vi "SpikeMIDI.vi"() -> ()   [LabVIEW 2022 SP3]
uses:
  _LVsubs/MakeYourOwn/Serial_Port.xctl
  _LVsubs/MakeYourOwn/Code.xctl
  _LVsubs/MakeYourOwn/File Tree.xctl
panel:
  in  "sensor 6":u16(ring)=1 items=["", "Touch Sensor", "Color Sensor", "Force and Distance", "Color and Distance", "Force and Motor", "Color and Motor"]
  in  "Port 7":string="A"
  in  "port 6":string="F"
  in  "six notes":bool
  in  "note (input a number) 6":string="70"
  in  "sensor 5":u16(ring)=1 items=["", "Touch Sensor", "Color Sensor", "Force and Distance", "Color and Distance", "Force and Motor", "Color and Motor"]
  in  "Port 6":string="B"
  in  "port 5":string="E"
  in  "five notes":bool
  in  "note (input a number) 5":string="70"
  in  "sensor 4":u16(ring)=1 items=["", "Touch Sensor", "Color Sensor", "Force and Distance", "Color and Distance", "Force and Motor", "Color and Motor"]
  in  "Port 5":string="C"
  in  "port 4":string="D"
  in  "four notes":bool
  in  "note (input a number) 4":string="70"
  in  "sensor 3":u16(ring)=1 items=["", "Touch Sensor", "Color Sensor", "Force and Distance", "Color and Distance", "Force and Motor", "Color and Motor"]
  in  "Port 4":string="D"
  in  "port 3":string="C"
  in  "three notes":bool
  in  "note (input a number) 3":string="70"
  in  "sensor 2":u16(ring)=1 items=["", "Touch Sensor", "Color Sensor", "Force and Distance", "Color and Distance", "Force and Motor", "Color and Motor"]
  in  "Port 3":string="E"
  in  "port 2":string="B"
  in  "two notes":bool
  in  "note (input a number) 2":string="70"
  in  "Port 2":string="F"
  in  "Port":string="A"
  in  "note (input a number)":string="60"
  in  "sensor":u16(ring)=1 items=["", "Touch Sensor", "Color Sensor", "Force and Distance", "Color and Distance", "Force and Motor", "Color and Motor"]
  in  "music":bool
  in  "MIDI Setup":bool
  in  "midi name (max 8 characters)":string="MIDI"
  out "BLE Good?":bool
  in  "BLE":bool
  in  "Serial_Port":T2(xcontrol)={"session"=refnum, "PyPath"=path "C:/Users/abbie/OneDrive/Desktop/ME35_21-main4/ME35_21-main/PythonIDE/_LVsubs/Serial/RogersSerial.py", "Processor"=enum."SPIKE", "Port"="COM18", "version"="3.7"}
  in  "Stop":bool
  in  "Settings":bool
  out "good?":bool
  in  "version":bool
  in  "reconnect":bool
  in  "Spike":bool
  in  "CtrlE":bool
  in  "Send Code":bool
  in  "Tab Control":enum32{"Chart", "Scope", "Last lines"}(tab)
  out "Chart":dbl(graph)=275.0
  out "Graph":dbl[](graph)
  in  "new lines":string[](array[string])=[">>> \r"]
  out "concatenated string":string="from ble_emma import *\nfrom ble_MIDI import *\nwhile not done():\n    if Force_Sensor_Activated(port.D):\n        play_note(\"m\", 60, .5, 'ffff',port.A)\ndisconnect()"
  in  "Console":string="\n>>> \n>>> \n>>> "
  in  "Path":path
  in  "Code":string(xcontrol)
  in  "File Tree":path(xcontrol)=path "C:/Users/abbie/OneDrive/Desktop/ME35_21-main4/ME35_21-main/PythonIDE/codes/test.py"
  # "Step 1: Choose the Spike as your Serial Port"
  # "step 2: hit the run button in the top left corner"
  # "step 3: set up bluetooth/midi"
  # "step 4: program an instrument!"
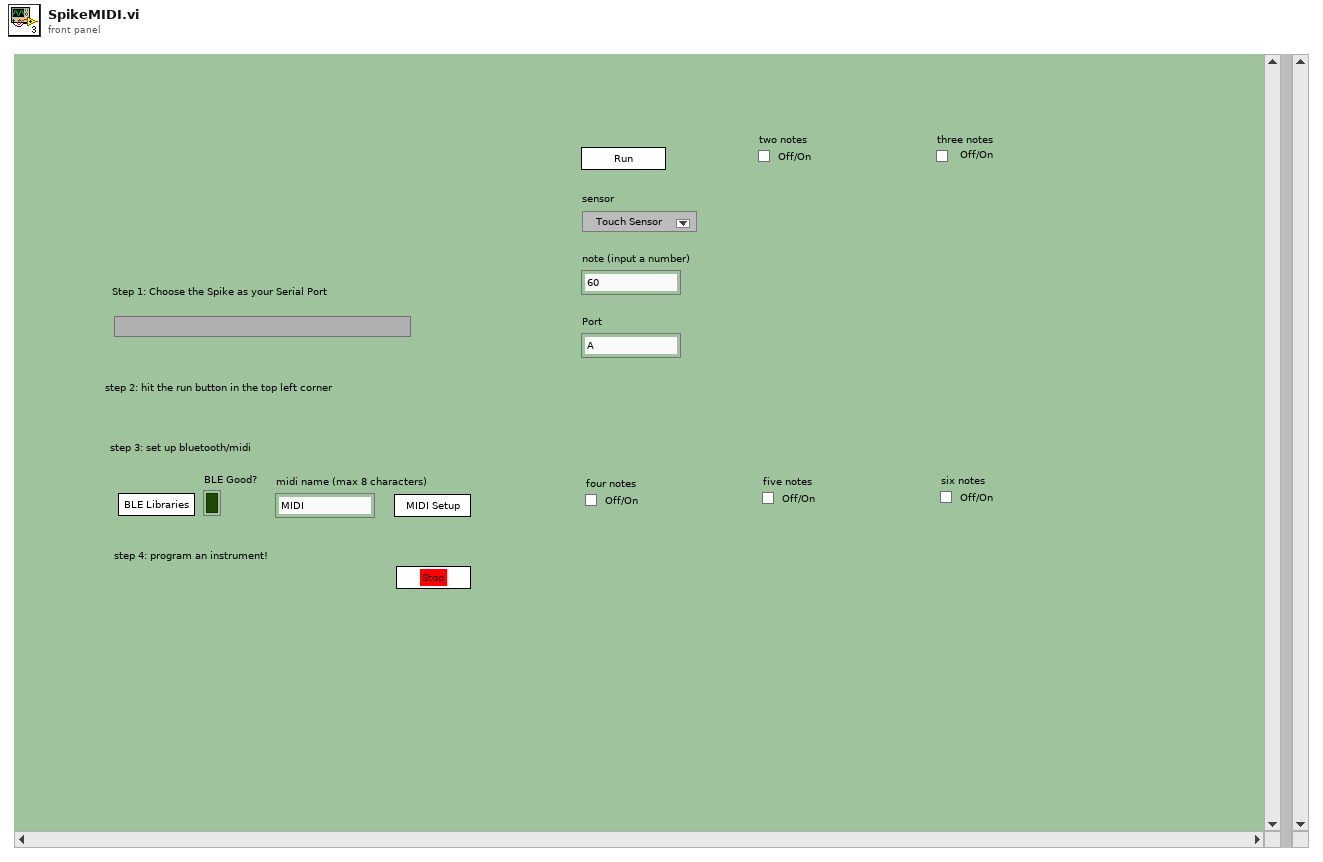
[diagram p1: front panel]
types:
  T1 = typedef "Processors.ctl" = enum16{"SPIKE", "Pi", "Pi_ssh", "OpenMV", "Dunio"}
  T2 = cluster{"session":refnum<k35>, "PyPath":path, "Processor":T1, "Port":string, "version":string}
  T3 = typedef "Preferences.ctl" = cluster{"python":string, "arduino CLI":path, "pythonCodes":cluster{"pythonCode":path, "Color":u32}[], "FontSize":u8, "Text Colors":cluster{"Quote":u32, "function":u32, "Python":u32, "Comment":u32, "Triple Quote":u32, "Text":u32}, "SSH Logins":cluster{"IP Address":string, "Username":string, "password":string}[], "packet size":u8}
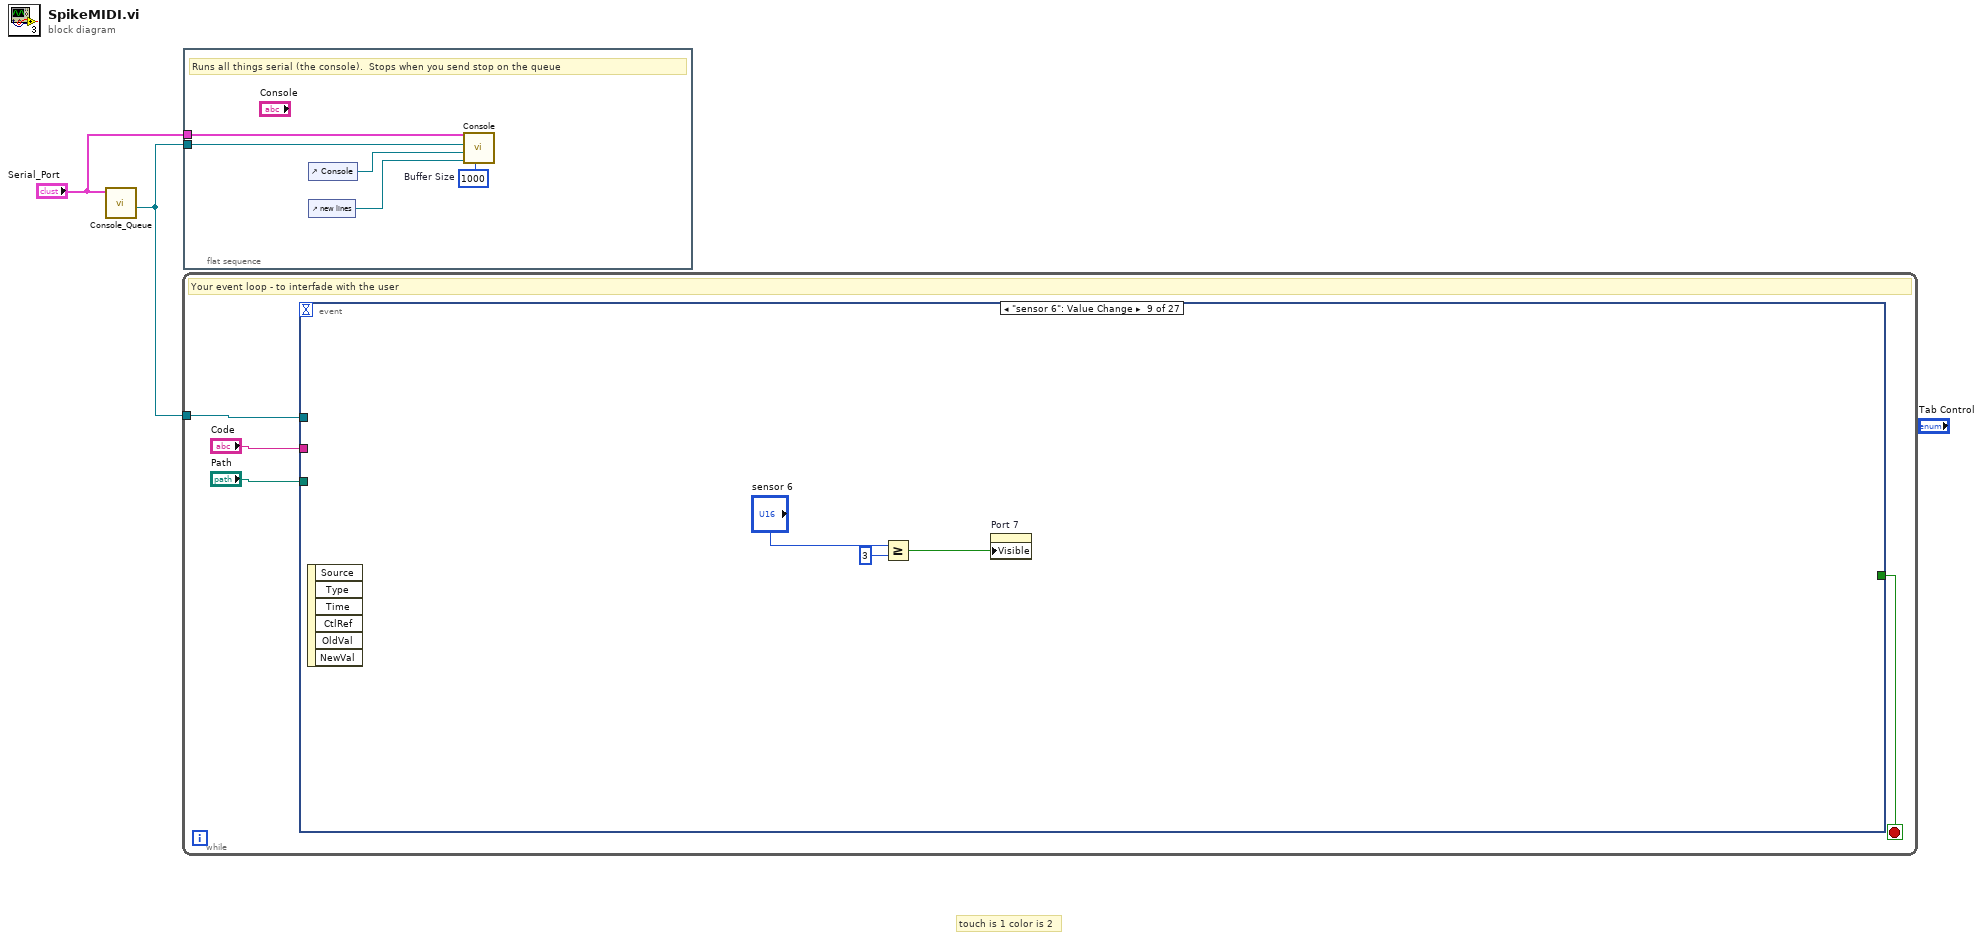
[diagram p0: block diagram]
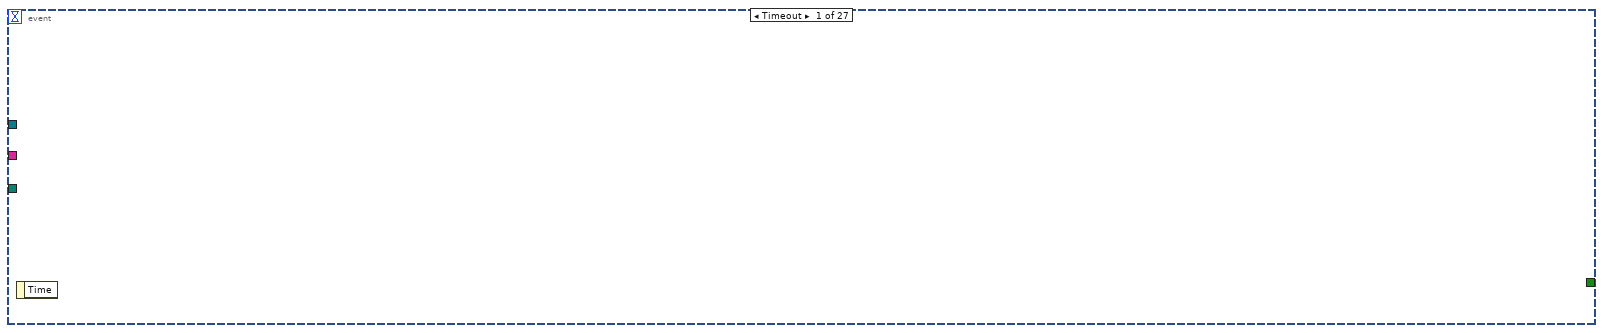
[diagram p2: hidden frame]
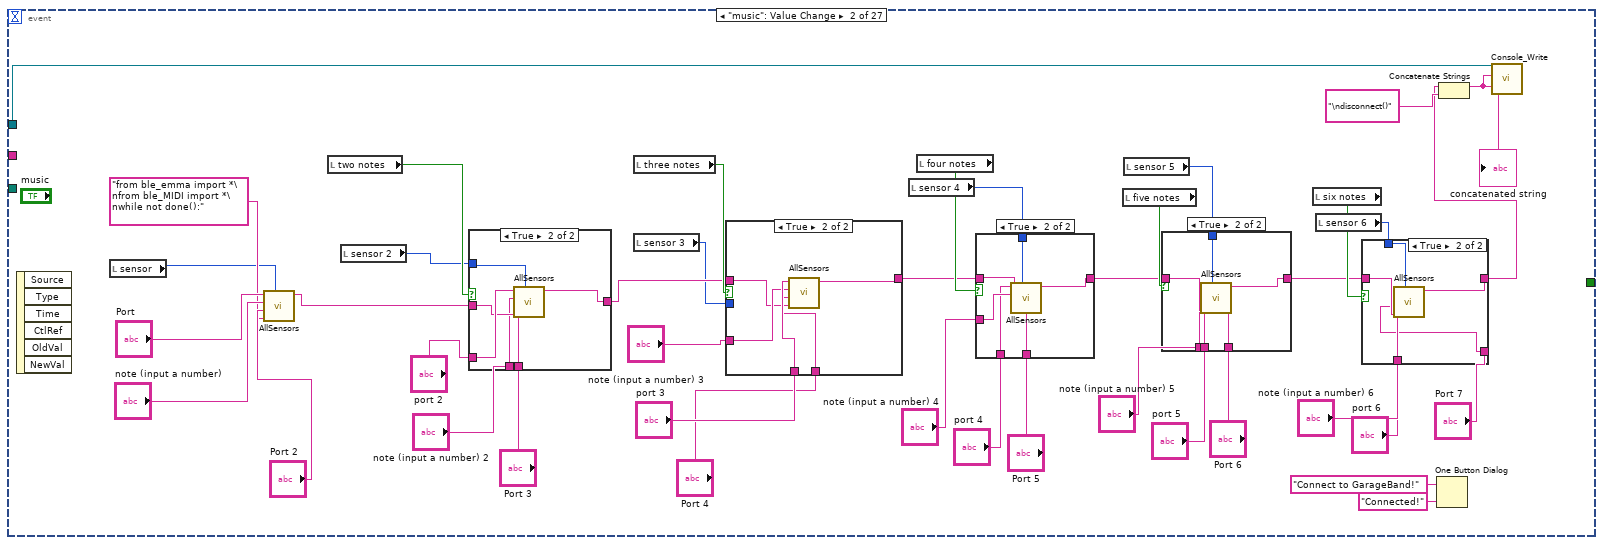
[diagram p3: hidden frame]
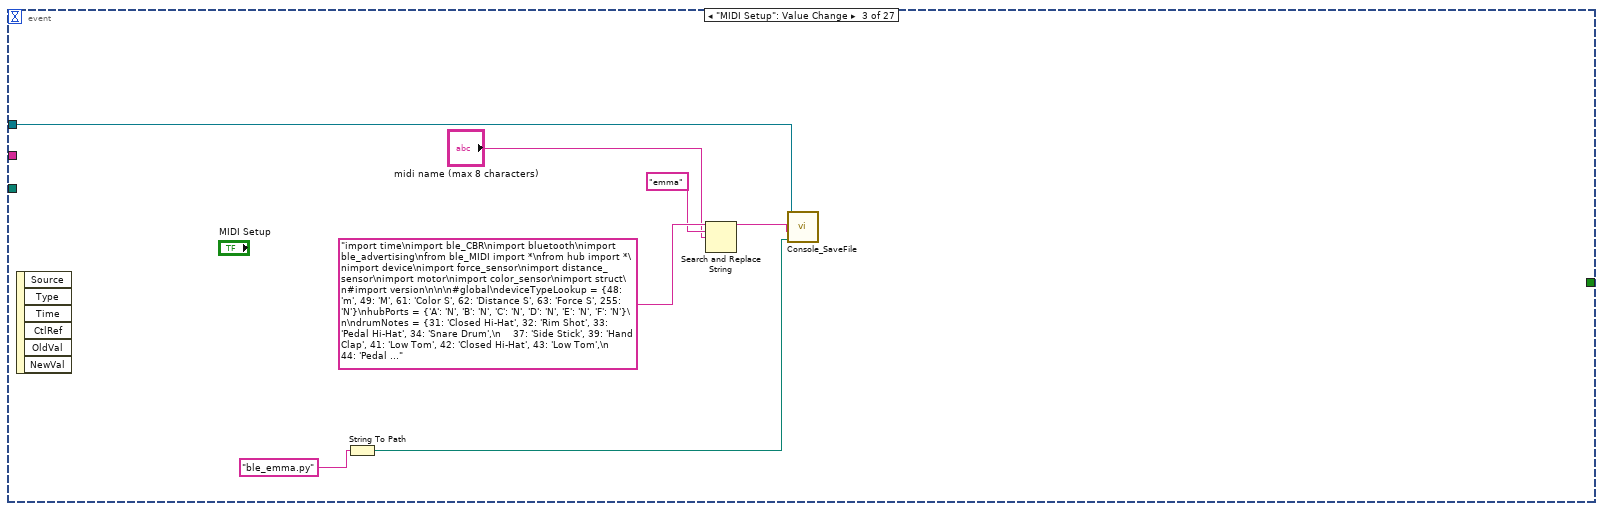
[diagram p9: hidden frame]
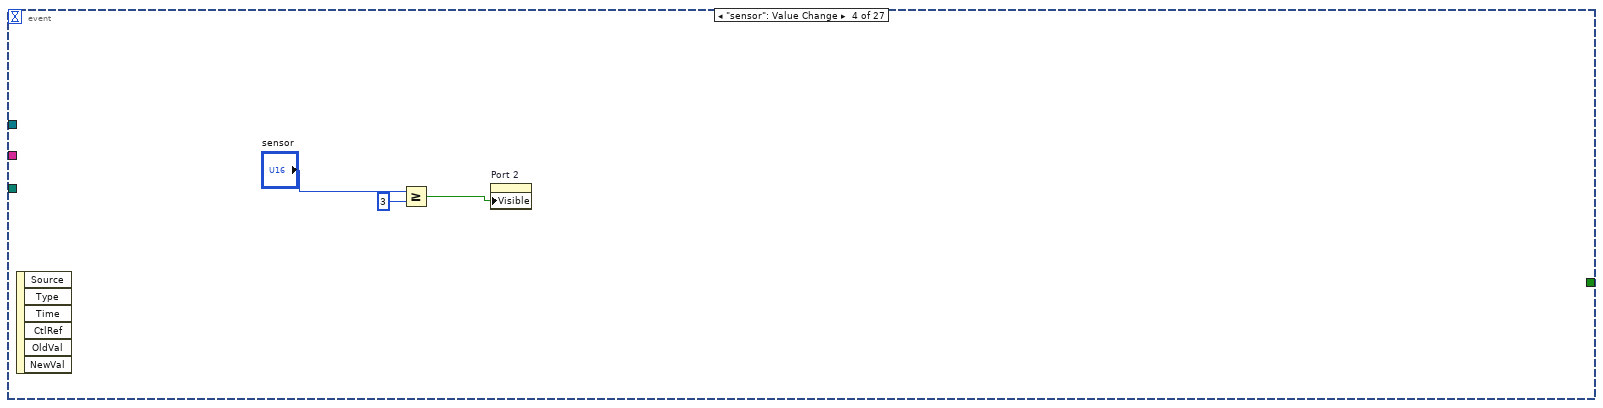
[diagram p10: hidden frame]
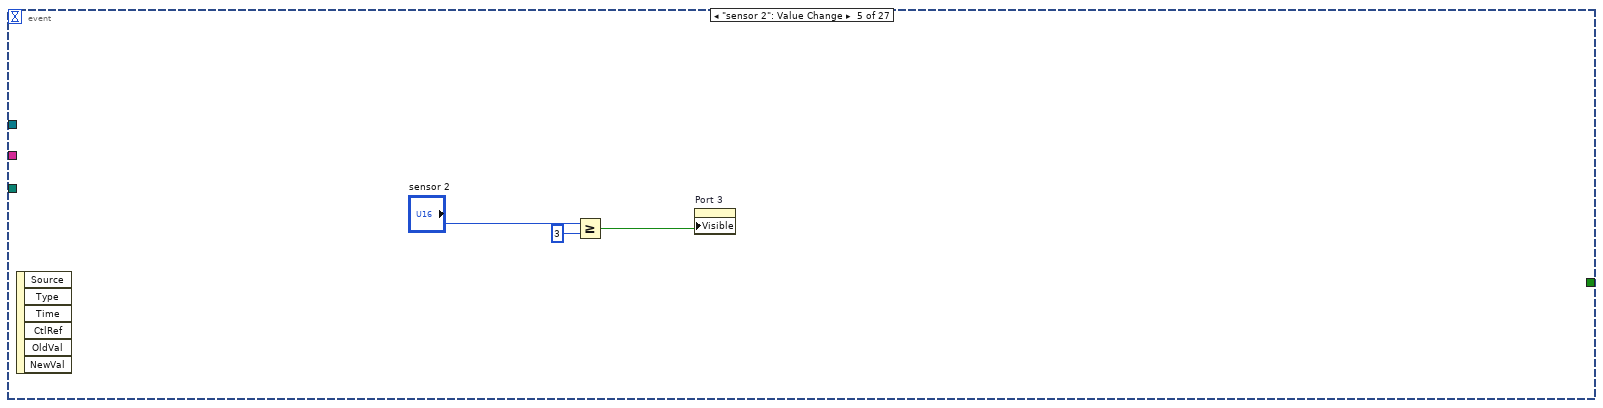
[diagram p11: hidden frame]
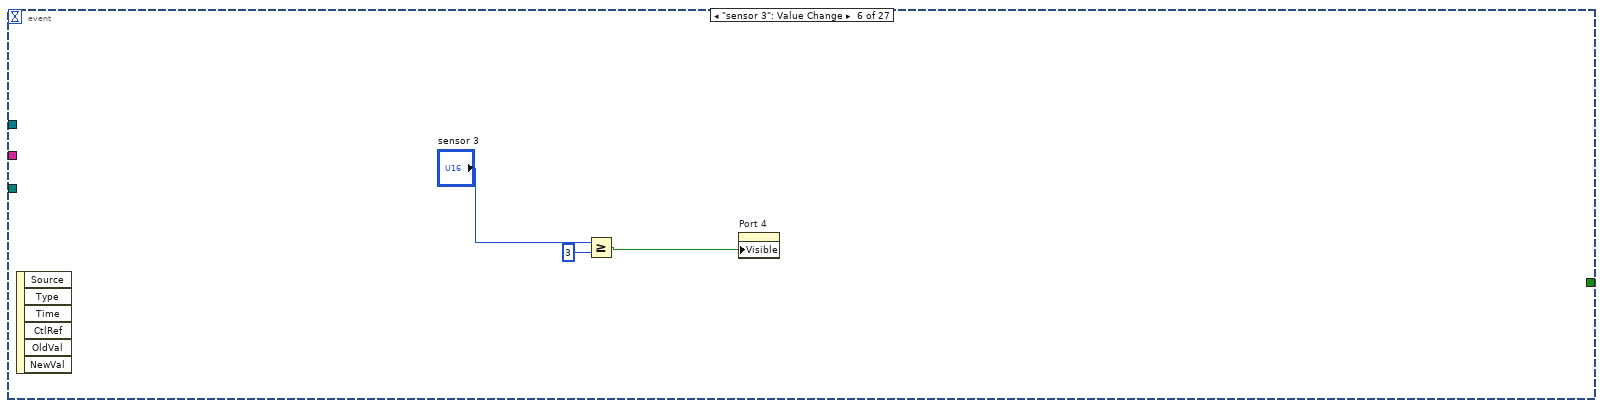
[diagram p12: hidden frame]
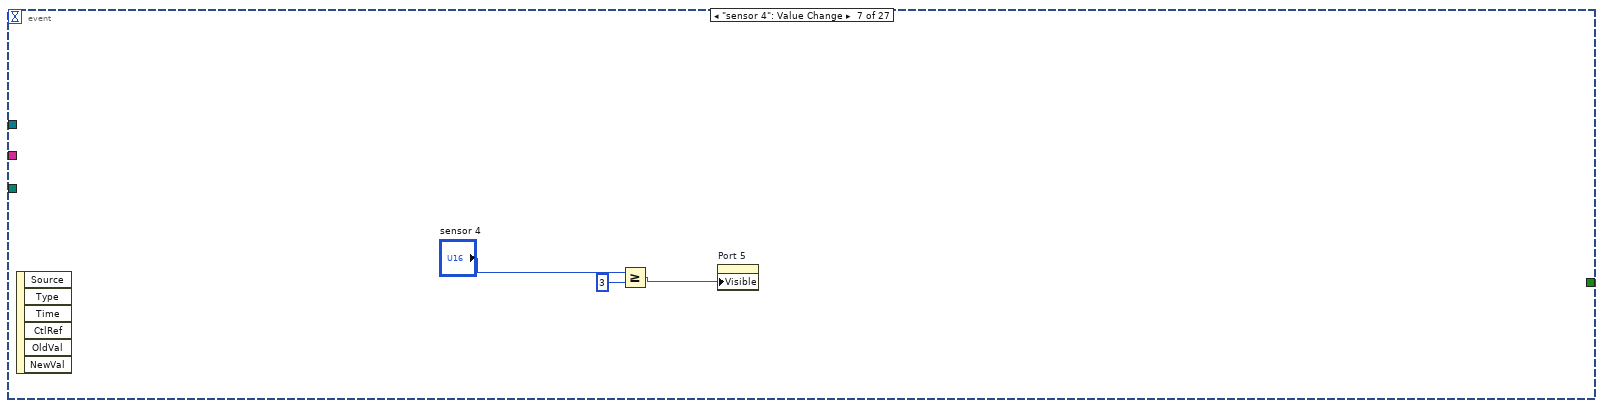
[diagram p13: hidden frame]
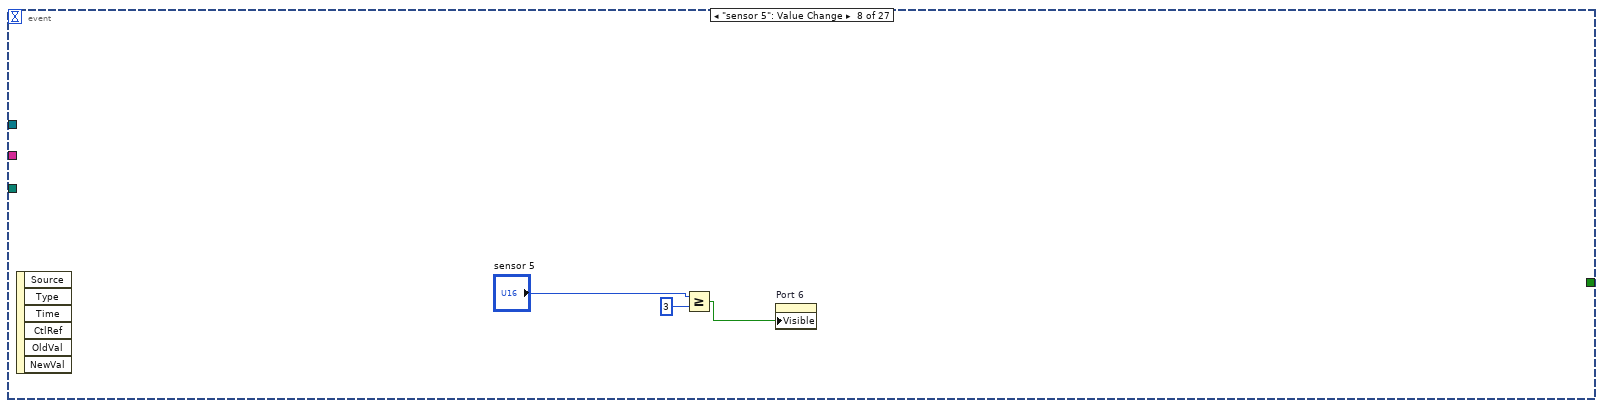
[diagram p14: hidden frame]
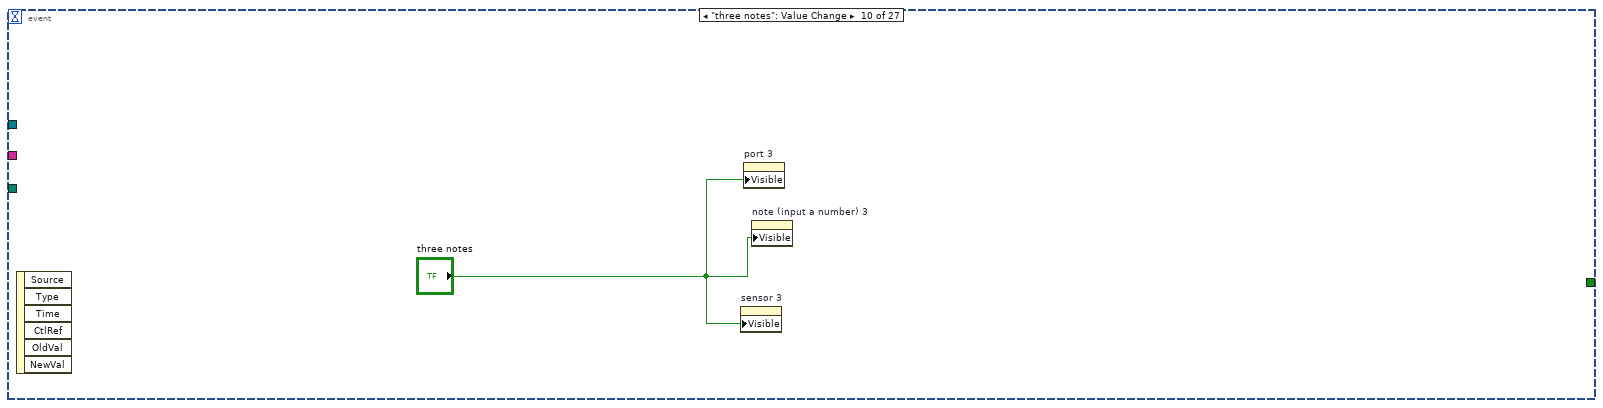
[diagram p15: hidden frame]
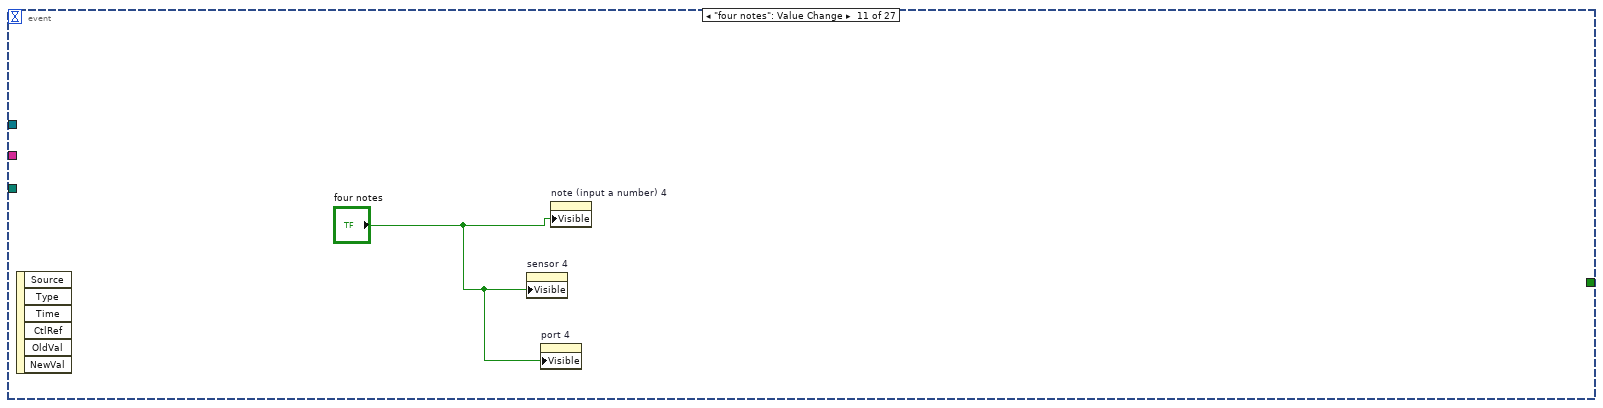
[diagram p16: hidden frame]
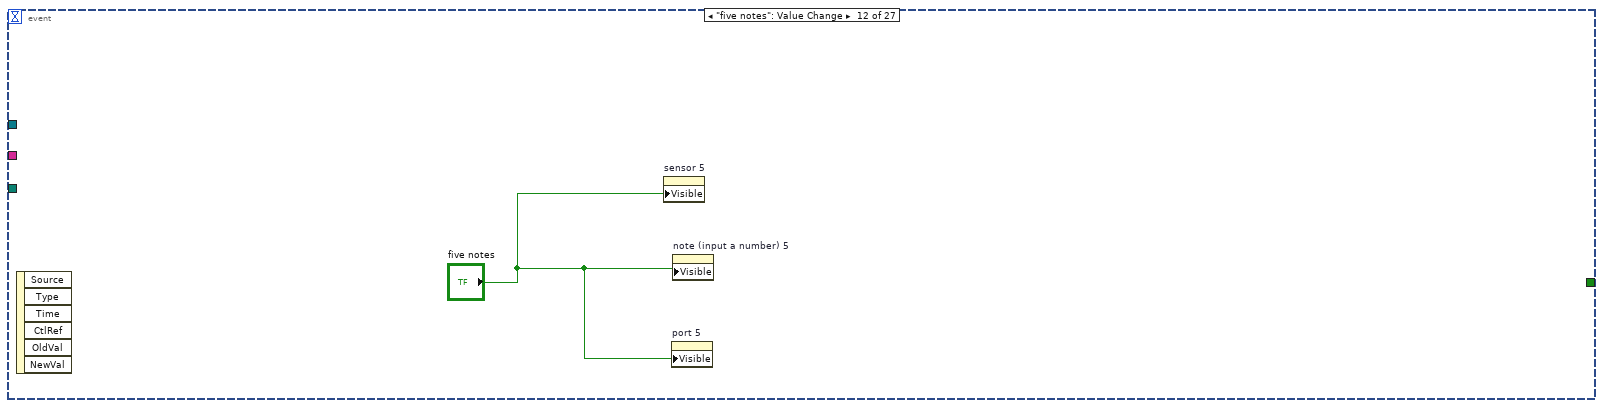
[diagram p17: hidden frame]
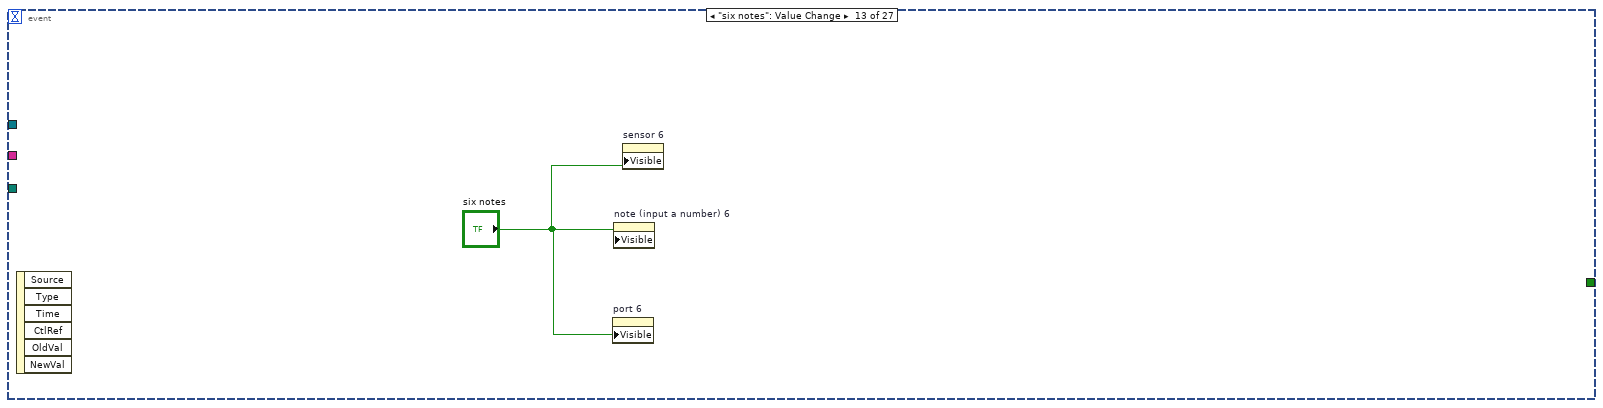
[diagram p18: hidden frame]
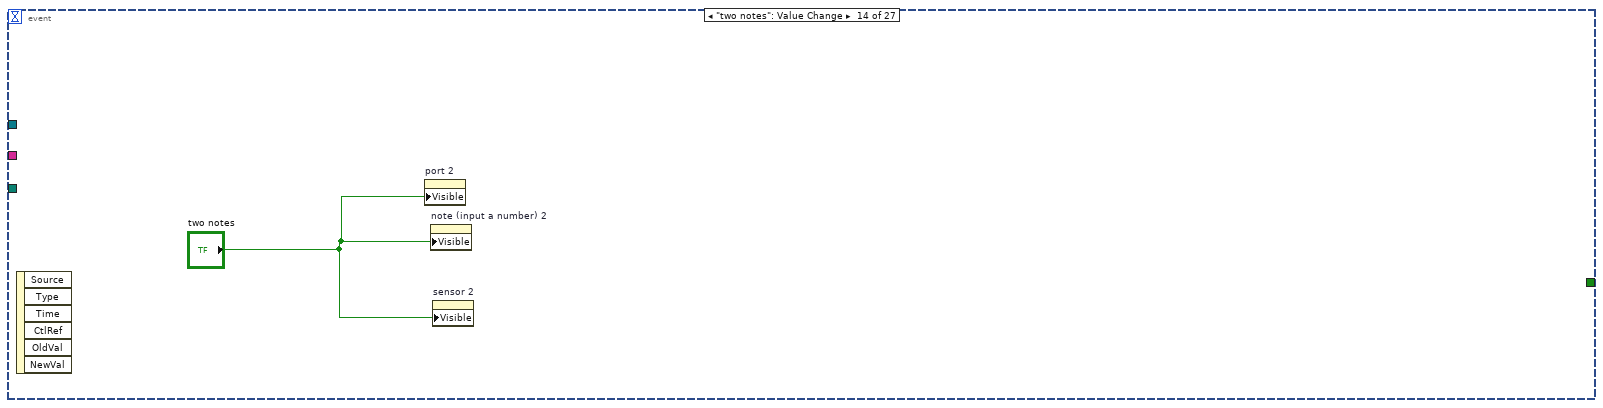
[diagram p19: hidden frame]
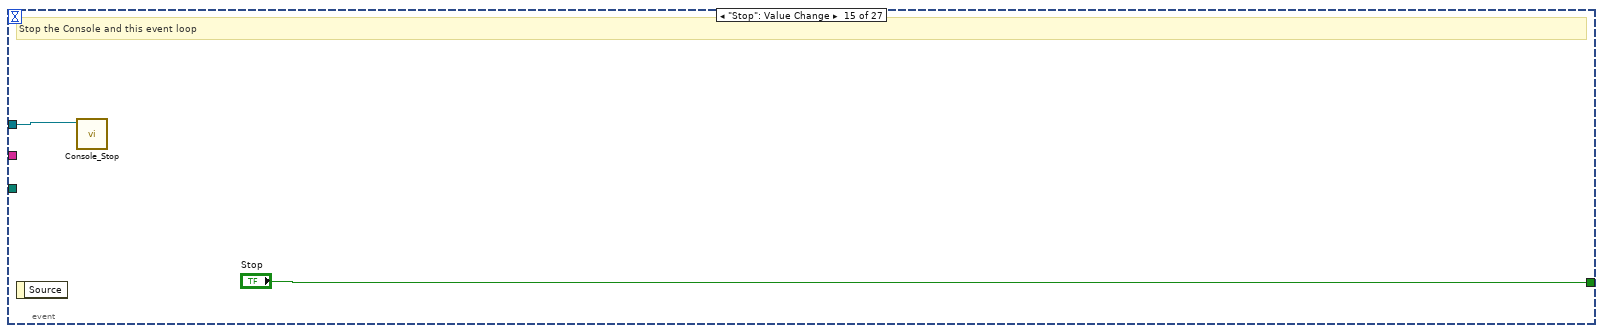
[diagram p20: hidden frame]
diagram:
  # "touch is 1 color is 2"
  n1 = call "Console_Queue.vi"("Serial_Port"="Serial_Port") -> ("Queue out"=w2:refnum<queue>)  [unwired: 9 in, 1 out]
  n2 = while {
    tunnel: w2 -> [w5]
    stop <- w6 stop-if-true
    # "Your event loop - to interfade with the user"
    n3 = event shown="[8] \"sensor 6\": Value Change" {
      selector: _ -> [_ _ _ _ _ _ _ _ _ _ _ _ _ _ _ _ _ _ _ _ _ _ _ _ _ _ _]
      dyn-events: _ -> [_ _ _ _ _ _ _ _ _ _ _ _ _ _ _ _ _ _ _ _ _ _ _ _ _ _ _]
      timeout: _ -> [_ _ _ _ _ _ _ _ _ _ _ _ _ _ _ _ _ _ _ _ _ _ _ _ _ _ _]
      tunnel: [_ _ _ _ _ _ _ _ _ _ _ _ _ _ "Stop" w115 _ _ _ _ _ _ _ _ _ _ _] -> w6
      tunnel: w5 -> [_ w47 w82 _ _ _ _ _ _ _ _ _ _ _ w112 w114 _ _ _ w128 w130 w131 w134 w137 w138 _ w140]
      tunnel: "Path" -> [_ _ _ _ _ _ _ _ _ _ _ _ _ _ _ _ _ _ w122 _ _ _ _ w135 _ _ _]
      tunnel: "Code" -> [_ _ _ _ _ _ _ _ _ _ _ _ _ _ _ _ _ _ _ w127 _ _ w133 w136 _ _ _]
      event Timeout {
        n4 = event-data() -> ()  [unwired: 1 in, 1 out]
      }
      event "music": Value Change {
        n5 = event-data() -> ()  [unwired: 1 in, 6 out]
        n6 = local read "sensor"() -> (w32:u16)
        n7 = call "AllSensors.vi"("sensor"=w32, "String in"="from ble_emma import *\nfrom ble_MIDI import *\nwhile not done():", "Port 2"="Port 2", "note (input a number)"="note (input a number)", "Port"="Port") -> ("String out"=w31:string)  [unwired: 6 in]
        n8 = local read "two notes"() -> (w41:bool)
        n9 = local read "sensor 2"() -> (w27:u16)
        n10 = case shown="True" w41 {
          tunnel: "port 2" -> [_ w79]
          tunnel: w27 -> [_ w80]
          tunnel: [w75 w81] -> w39
          tunnel: w31 -> [w75 w78]
          tunnel: "note (input a number) 2" -> [_ w77]
          tunnel: "Port 3" -> [_ w76]
          frame False {
          }
          frame True {
            n11 = call "AllSensors.vi"("sensor"=w80, "String in"=w78, "Port 2"=w76, "note (input a number)"=w77, "Port"=w79) -> ("String out"=w81:string)  [unwired: 6 in]
          }
        }
        n12 = local read "three notes"() -> (w40:bool)
        n13 = local read "sensor 3"() -> (w26:u16)
        n14 = case shown="True" w40 {
          tunnel: w39 -> [w69 w70]
          tunnel: [w69 w74] -> w22
          tunnel: "note (input a number) 3" -> [_ w72]
          tunnel: w26 -> [_ _]
          tunnel: "port 3" -> [_ w73]
          tunnel: "Port 4" -> [_ w71]
          frame False {
          }
          frame True {
            n15 = call "AllSensors.vi"("String in"=w70, "Port 2"=w71, "note (input a number)"=w72, "Port"=w73) -> ("String out"=w74:string)  [unwired: 7 in]
          }
        }
        n16 = local read "sensor 4"() -> (w18:u16)
        n17 = local read "four notes"() -> (w25:bool)
        n18 = case shown="True" w25 {
          tunnel: w22 -> [w62 w64]
          tunnel: [w62 w63] -> w21
          tunnel: w18 -> [_ w68]
          tunnel: "note (input a number) 4" -> [_ w67]
          tunnel: "port 4" -> [_ w66]
          tunnel: "Port 5" -> [_ w65]
          frame False {
          }
          frame True {
            n19 = call "AllSensors.vi"("sensor"=w68, "String in"=w64, "Port 2"=w65, "note (input a number)"=w67, "Port"=w66) -> ("String out"=w63:string)  [unwired: 6 in]
          }
        }
        n20 = local read "five notes"() -> (w24:bool)
        n21 = local read "sensor 5"() -> (w17:u16)
        n22 = case shown="True" w24 {
          tunnel: w21 -> [w55 w60]
          tunnel: [w55 w59] -> w20
          tunnel: w17 -> [_ w61]
          tunnel: "note (input a number) 5" -> [_ w58]
          tunnel: "port 5" -> [_ w57]
          tunnel: "Port 6" -> [_ w56]
          frame False {
          }
          frame True {
            n23 = call "AllSensors.vi"("sensor"=w61, "String in"=w60, "Port 2"=w56, "note (input a number)"=w58, "Port"=w57) -> ("String out"=w59:string)  [unwired: 6 in]
          }
        }
        n24 = local read "six notes"() -> (w23:bool)
        n25 = local read "sensor 6"() -> (w16:u16)
        n26 = case shown="True" w23 {
          tunnel: w20 -> [w48 w53]
          tunnel: [w48 w52] -> w19
          tunnel: w16 -> [_ w54]
          tunnel: "note (input a number) 6" -> [_ w51]
          tunnel: "port 6" -> [_ w50]
          tunnel: "Port 7" -> [_ w49]
          frame False {
          }
          frame True {
            n27 = call "AllSensors.vi"("sensor"=w54, "String in"=w53, "Port 2"=w49, "note (input a number)"=w51, "Port"=w50) -> ("String out"=w52:string)  [unwired: 6 in]
          }
        }
        n28 = One Button Dialog(message="Connect to GarageBand!", button name ("OK")="Connected!") -> ()  [unwired: 1 out]
        n29 = Concatenate Strings(w19, "\ndisconnect()" ("string")) -> (w42:string)
        "concatenated string" <- w42
        n30 = call "Console_Write.vi"("Code"=w42, "Queue in"=w47) -> ()  [unwired: 10 in]
      }
      event "MIDI Setup": Value Change {
        n31 = event-data() -> ()  [unwired: 1 in, 6 out]
        n32 = String To Path(string="ble_emma.py") -> (path=w85:path)
        n33 = Search and Replace String(input string="import time\nimport ble_CBR\nimport bluetooth\nimport ble_advertising\nfrom ble_MIDI import *\nfrom hub import *\nimport device\nimport force_sensor\nimport distance_sensor\nimport motor\nimport color_sensor\nimport struct\n#import version\n\n\n#global\ndeviceTypeLookup = {48: 'm', 49: 'M', 61: 'Color S', 62: 'Distance S', 63: 'Force S', 255: 'N'}\nhubPorts = {'A': 'N', 'B': 'N', 'C': 'N', 'D': 'N', 'E': 'N', 'F': 'N'}\n\ndrumNotes = {31: 'Closed Hi-Hat', 32: 'Rim Shot', 33: 'Pedal Hi-Hat', 34: 'Snare Drum',\n    37: 'Side Stick', 39: 'Hand Clap', 41: 'Low Tom', 42: 'Closed Hi-Hat', 43: 'Low Tom',\n    44: 'Pedal Hi-Hat', 45: 'Mid Tom', 46: 'Open Hi-Hat', 47: 'Mid Tom', 48: 'High Tom',\n    49: 'Crash Cymbal', 50: 'High Tom', 51: 'Ride Cymbal', 52: 'Ride Cymbal', 53: 'Ride Bell',\n    54: 'Shaker', 57: 'Crash Cymbal', 59: 'Ride Cymbal', 86: 'Snare Drum', 90: 'Closed Hi-Hat',\n    91: 'Low Tom', 92: 'Closed Hi-Hat', 94: 'Pedal Hi-Hat', 95: 'Mid Tom',96: 'High Tom',\n    99: 'Ride Cymbal'}\n\n\n#firmware_check()\n\ndef done():\n    return button.pressed(button.RIGHT)\n\n\ndef test():\n    print(\"hi Emma!\")\n\n\ndef play_note(sensor = \"N\", note = 60, duration = 1, dynamics = 'fff', port = None):\n    \n    #print(\"in play_note\")\n\n    if type(note) == str:  \n        for key, value in drumNotes.items():\n            if value == note:\n                note = key  \n                #print(\"Found note:\", note)\n\n            \n    if (sensor == \"N\"):  \n        play_the_note(note, duration, dynamics)    \n        \n    elif (sensor == \"Force S\"):\n        if Force_Sensor_Activated(port):\n            play_the_note(note, duration, dynamics)\n        else:\n            print(\"waiing for FS activation\")\n            time.sleep(.1)\n            \n    elif (sensor == \"Color S\"):\n        if Color_Sensor_Activated(port):\n            play_the_note(note, duration, dynamics)\n        else:\n            print(\"waiting for CS activation\")\n            time.sleep(.1)\n            \n    elif (sensor == \"Distance S\"):\n        if Distance_Sensor_Activated(port):\n            #the_ports = check_port_connection(\"Distance S\")\n            #for port in the_ports:\n            if distance_sensor.distance(port) > 0:\n                dist = distance_sensor.distance(port)\n                dist_note = get_note_from_distance(dist)\n                play_the_note(dist_note, duration, dynamics)\n            #play_the_note(note, duration)\n        else:\n            print(\"waiting for DS activation\")\n            time.sleep(.1)\n            \n    elif ((sensor == \"m\") or (sensor == \"M\")):\n        #Need and if activated statment bc it could be not conencted\n        #the_ports = check_port_connection(\"m\")\n        #for port in the_ports:\n        note_value = motor_pos(port)\n        play_the_note(note_value, duration, dynamics)\n        \n    else: \n        print(\"ELSE!!Invalid sensor type\")\n        time.sleep(.5)       \n\n\ndef play_chord(a, b=0, c=0, d=0, e=0, f=0, g=0, h=0):\n    Piano.on([a,b,c,d,e,f,g,h],velocity['ff'])\n    time.sleep(.5)\n    Piano.off([a,b,c,d,e,f,g,h])\n        \n        \ndef play_the_note(note, duration, dynamics):\n    Piano.on(note, velocity[dynamics])\n    time.sleep(duration)\n    Piano.off(note, velocity[dynamics])\n\n\ndef Force_Sensor_Activated(port):\n    try:\n        if port is None:\n            the_ports = check_port_connection(\"Force S\")\n            if the_ports is None:\n                #print(\"Please connect the Force Sensor!\")\n                raise Exception(\"Force Sensor is NOT connected\")\n            \n            for port in the_ports:\n                if force_sensor.force(port) > 0:\n                    print(\"Force Sensor is ACTIVATED\")\n                    return True\n            \n            return False\n        else:\n            try:\n                if force_sensor.force(port) > 0:\n                    print(\"Force Sensor is ACTIVATED\")\n                    return True\n                else:\n                    #print(\"FS FALSE\")\n                    #time.sleep(.25)\n                    return False\n            except:\n                print(\"Error: Force Sensor is NOT connected in the right port\")\n                time.sleep(2)\n                return False\n                \n                        \n    except Exception as e:\n        print(f\"Error: {e}\")\n        time.sleep(2)\n        return False\n\n\n    \ndef Color_Sensor_Activated(port):\n    try:\n        if port is None:\n            the_ports = check_port_connection(\"Color S\")\n            if the_ports is None:\n                #print(\"Please connect the Color Sensor!\")\n                raise Exception(\"Color Sensor is NOT connected\")\n            \n            for port in the_ports:\n                if color_sensor.reflection(port) > 50:\n                    print(\"Color Sensor is ACTIVATED\")\n                    return True\n            \n            return False\n        else:\n            try:\n                if color_sensor.reflection(port) > 50:\n                    print(\"Color Sensor is ACTIVATED\")\n                    return True\n                else:\n                    return False\n                    \n            except:\n                print(\"Error: Color Sensor is NOT connected in the right port\")\n                time.sleep(2)\n                return False\n                    \n    except Exception as e:\n        print(f\"Error: {e}\")\n        time.sleep(2)\n        return False\n\n        \ndef Distance_Sensor_Activated(port):\n    try:\n        if port is None:\n            the_ports = check_port_connection(\"Distance S\")\n            if the_ports is None:\n                #print(\"Please connect the Color Sensor!\")\n                raise Exception(\"Distance Sensor is NOT connected\")\n            \n            for port in the_ports:\n                if distance_sensor.distance(port) > 0:\n                    print(\"Distance Sensor is ACTIVATED\")\n                    return True\n\n            return False\n        else:\n            try:\n                if distance_sensor.distance(port) > 0:\n                    print(\"Distance Sensor is ACTIVATED\")\n                    return True\n                else:\n                    return False\n                    \n            except: \n                print(\"Error: Distance Sensor is NOT connected in the right port\")\n                time.sleep(2)\n                return False\n        \n    except Exception as e:\n        print(f\"Error: {e}\")\n        time.sleep(2)\n        return False    \n\n\n'''\ndef Motor_Activated(port):\n    try:\n        if port is None:\n            the_ports = check_port_connection(\"m\")\n            if the_ports is None:\n                raise Exception(\"small motor is NOT connected\")\n            \n            for port in the_ports:\n                motor_pos(port)\n                print(\"small motor is ACTIVATED\")\n                return True\n\n        else:\n            if distance_sensor.distance(port) > 0:\n                print(\"Distance Sensor is ACTIVATED\")\n                return True\n            else:\n                return False\n\n    except Exception as e:\n        print(f\"Error: {e}\")\n        time.sleep(2)\n        return False    \n'''\n\ndef motor_pos(port):  \n    try:\n        mpos = motor.absolute_position(port)\n                \n        if mpos < 0:\n            mpos = mpos + 360  \n                    \n        print(mpos)\n        note_range = 108 - 21  #Total number of notes in the range\n        note_value = int((mpos / 360) * note_range) + 21  #Maps the notes and value\n        \n        return note_value\n        \n    except:\n        print(\"Error: Motor is NOT connected in the right port\")\n        time.sleep(2)\n        return False\n\n\n\ndef disconnect():\n    print('disconnect')\n    midi.disconnect()\n\n\n\n\ndef NoteToNumber(note, octave = 0):\n    notes = {\"C\": 24,\"Db\": 25,\"D\": 26,\"Eb\": 27,\"E\": 28,\"F\": 29,\"Gb\": 30,\"G\": 31,\"Ab\": 32, \"A\": 33,\"Bb\": 34,\"B\": 35}\n    \n    try:  \n        if octave > 8 or octave < 0:\n            raise Exception(\"Invalid octave input\")\n        if note not in notes:\n            raise Exception(\"Invalid note input\")\n    \n        if(octave > 0):\n            return((notes[note]) + (octave*12))\n        \n    except Exception as e:\n        print(f\"Error: {e}\")\n        time.sleep(2)\n        return False\n        \n    \n'''-----Helper functions section (NOT intended for the user to use!)-----'''\n'''\ndef firmware_check():\n    try:\n        version.atlantis\n        print(version.atlantis)\n        print(\"Firmware is up to date! Good Job!\")\n    except:\n        print(\"Old Firmware: Please update your LEGO SPIKE hub to the latest firmware!\")\n'''\n\ndef get_note_from_distance(dist):\n    if dist == -1 or dist > 500:\n        return -1\n    elif dist < 500:\n        note = int(8 + (dist / 5))\n        return note\n\n\n\ndef ReadPorts(self):\n    for i in range(6):\n        if device.ready(i):\n            self.deviceType[i] = deviceTypeLookup[device.id(i)]\n        else:\n            self.deviceType[i] = None\n            \ndef is_connected(sensor):\n    ReadPorts()\n    \n    there_is_sensor = False\n    \n    i = 0\n    for port in sorted(hubPorts):\n        \n        if hubPorts[port] == sensor:\n            print(f\"{sensor} is connected to port.{port}\")\n            there_is_sensor = True\n    \n        if i == 5 and not there_is_sensor:\n            print(f\"{sensor} is NOT connected\")\n            print(\"--------------\")\n            raise ValueError(f\"{sensor} is not connected to any port\")\n            return False\n            \n        if i == 5 and there_is_sensor:\n            return True\n            \n        i+=1\n\n    return False\n\n\ndef check_port_connection(sensor):\n    ReadPorts()\n    listOfPorts = []\n    is_a_connection = False\n    i = 0\n    for port in sorted(hubPorts):\n        \n        if hubPorts[port] == sensor:      \n            listOfPorts.append(string2port(f\"port.{port}\"))\n            is_a_connection = True\n            #return string2port(f\"port.{port}\")\n            #return(f\"port.{port}\")\n    \n        if i == 5 and is_a_connection:\n            #print(listOfPorts)\n            return listOfPorts\n            \n            \n        if i == 5 and not is_a_connection:\n            print(f\"{sensor} is NOT connected\")\n            print(\"--------------\")\n            #raise Exception(f\"{sensor} is NOT connected\")\n            return None\n        \n        i+=1\n    \n    return None\n        \n    \ndef string2port(portS):\n    if portS == \"port.A\": return port.A\n    if portS == \"port.B\": return port.B\n    if portS == \"port.C\": return port.C\n    if portS == \"port.D\": return port.D\n    if portS == \"port.E\": return port.E\n    if portS == \"port.F\": return port.F\n\n\n\n#initialize\nmidi = MIDI_Player('emma')\nmidi.wait_for_connection()\nPiano = MIDI_Instrument(midi, instruments['Acoustic Grand Piano'], channel=0)\n", search string="emma", replace string="midi name (max 8 characters)") -> (result string=w84:string)  [unwired: 5 in, 3 out]
        n34 = call "Console_SaveFile.vi"("Path"=w85, "Code"=w84, "Queue in"=w82) -> ()  [unwired: 9 in]
      }
      event "sensor": Value Change {
        n35 = event-data() -> ()  [unwired: 1 in, 6 out]
        n36 = Greater Or Equal?(x="sensor", y=u16 3) -> (x >= y?=w89:bool)
        n37 = property on="Port 2" class="Str"("Visible"=w89) -> ()  [unwired: 2 in, 2 out]
      }
      event "sensor 2": Value Change {
        n38 = event-data() -> ()  [unwired: 1 in, 6 out]
        n39 = Greater Or Equal?(x="sensor 2", y=u16 3) -> (x >= y?=w92:bool)
        n40 = property on="Port 3" class="Str"("Visible"=w92) -> ()  [unwired: 2 in, 2 out]
      }
      event "sensor 3": Value Change {
        n41 = event-data() -> ()  [unwired: 1 in, 6 out]
        n42 = Greater Or Equal?(x="sensor 3", y=u16 3) -> (x >= y?=w95:bool)
        n43 = property on="Port 4" class="Str"("Visible"=w95) -> ()  [unwired: 2 in, 2 out]
      }
      event "sensor 4": Value Change {
        n44 = event-data() -> ()  [unwired: 1 in, 6 out]
        n45 = Greater Or Equal?(x="sensor 4", y=u16 3) -> (x >= y?=w98:bool)
        n46 = property on="Port 5" class="Str"("Visible"=w98) -> ()  [unwired: 2 in, 2 out]
      }
      event "sensor 5": Value Change {
        n47 = event-data() -> ()  [unwired: 1 in, 6 out]
        n48 = Greater Or Equal?(x="sensor 5", y=u16 3) -> (x >= y?=w101:bool)
        n49 = property on="Port 6" class="Str"("Visible"=w101) -> ()  [unwired: 2 in, 2 out]
      }
      event "sensor 6": Value Change {
        n50 = event-data() -> ()  [unwired: 1 in, 6 out]
        n51 = Greater Or Equal?(x="sensor 6", y=u16 3) -> (x >= y?=w104:bool)
        n52 = property on="Port 7" class="Str"("Visible"=w104) -> ()  [unwired: 2 in, 2 out]
      }
      event "three notes": Value Change {
        n53 = event-data() -> ()  [unwired: 1 in, 6 out]
        n54 = property on="sensor 3" class="Ring (strict)"("Visible"="three notes") -> ()  [unwired: 2 in, 2 out]
        n55 = property on="port 3" class="Str"("Visible"="three notes") -> ()  [unwired: 2 in, 2 out]
        n56 = property on="note (input a number) 3" class="Str"("Visible"="three notes") -> ()  [unwired: 2 in, 2 out]
      }
      event "four notes": Value Change {
        n57 = event-data() -> ()  [unwired: 1 in, 6 out]
        n58 = property on="sensor 4" class="Ring (strict)"("Visible"="four notes") -> ()  [unwired: 2 in, 2 out]
        n59 = property on="port 4" class="Str"("Visible"="four notes") -> ()  [unwired: 2 in, 2 out]
        n60 = property on="note (input a number) 4" class="Str"("Visible"="four notes") -> ()  [unwired: 2 in, 2 out]
      }
      event "five notes": Value Change {
        n61 = event-data() -> ()  [unwired: 1 in, 6 out]
        n62 = property on="sensor 5" class="Ring (strict)"("Visible"="five notes") -> ()  [unwired: 2 in, 2 out]
        n63 = property on="port 5" class="Str"("Visible"="five notes") -> ()  [unwired: 2 in, 2 out]
        n64 = property on="note (input a number) 5" class="Str"("Visible"="five notes") -> ()  [unwired: 2 in, 2 out]
      }
      event "six notes": Value Change {
        n65 = event-data() -> ()  [unwired: 1 in, 6 out]
        n66 = property on="port 6" class="Str"("Visible"="six notes") -> ()  [unwired: 2 in, 2 out]
        n67 = property on="note (input a number) 6" class="Str"("Visible"="six notes") -> ()  [unwired: 2 in, 2 out]
        n68 = property on="sensor 6" class="Ring (strict)"("Visible"="six notes") -> ()  [unwired: 2 in, 2 out]
      }
      event "two notes": Value Change {
        n69 = event-data() -> ()  [unwired: 1 in, 6 out]
        n70 = property on="port 2" class="Str"("Visible"="two notes") -> ()  [unwired: 2 in, 2 out]
        n71 = property on="note (input a number) 2" class="Str"("Visible"="two notes") -> ()  [unwired: 2 in, 2 out]
        n72 = property on="sensor 2" class="Ring (strict)"("Visible"="two notes") -> ()  [unwired: 2 in, 2 out]
      }
      event "Stop": Value Change {
        # "Stop the Console and this event loop"
        n73 = event-data() -> ()  [unwired: 1 in, 1 out]
        n74 = call "Console_Stop.vi"("Queue in"=w112) -> ()  [unwired: 11 in]
      }
      event Panel Close? {
        w115 = TRUE ("Discard?")
        # "keep the window open"
        # "If they close the wondow - stop the program"
        n75 = event-data() -> ()  [unwired: 1 in, 1 out]
        n76 = call "Console_Stop.vi"("Queue in"=w114) -> ()  [unwired: 11 in]
        n77 = event-data("Discard?"=w115) -> ()  [unwired: 1 in, 1 out]
      }
      event "File Tree": Value Change {
        # "Put their selection into the path"
        n78 = event-data() -> ()  [unwired: 1 in, 1 out]
        n79 = property on="Path" class="Path"("Val(Sgnl)"="File Tree") -> ()  [unwired: 2 in, 2 out]
      }
      event "Path": Value Change {
        # "Open the chosen file"
        n80 = event-data() -> ("OldVal"=w119:path, "NewVal"=w117:path)  [unwired: 1 in]
        n81 = Not Equal?(x=w119, y=w117) -> (x != y?=w118:bool)
        n82 = case shown="False" w118 {
          tunnel: w117 -> [_ w121]
          frame False {
          }
          frame True {
            n83 = Read from Text File(file (use dialog)=w121) -> (text=w120:string)  [unwired: 3 in, 3 out]
            n84 = local write "Code"(w120) -> ()
          }
        }
      }
      event "Code": Value Change {
        # "save any changes they make"
        # "autosave code changes (if there is a file)"
        n85 = event-data() -> ("NewVal"=w124:string)  [unwired: 1 in]
        n86 = Empty String/Path?(string/path=w122) -> (empty?=w123:bool)
        n87 = case shown="False" w123 {
          tunnel: w124 -> [w126 _]
          tunnel: w122 -> [w125 _]
          frame False {
            n88 = Write to Text File(file (use dialog)=w125, text=w126) -> ()  [unwired: 2 in, 3 out]
          }
          frame True {
          }
        }
      }
      event "Send Code": Value Change {
        # "Run code in REPL"
        n89 = event-data() -> ()  [unwired: 1 in, 1 out]
        n90 = call "Console_Write.vi"("Code"=w127, "Queue in"=w128) -> ()  [unwired: 10 in]
      }
      event "version": Value Change {
        # "Run code in REPL"
        n91 = event-data() -> ()  [unwired: 1 in, 1 out]
        n92 = call "Console_Write.vi"("Code"="import version\n\ndef testVersion():\n    try:\n        version.atlantis\n        print('version good')\n    except:\n        print('version bad')\n        \ntestVersion()\n", "Queue in"=w130) -> ()  [unwired: 10 in]
      }
      event "BLE": Value Change {
        n93 = event-data() -> ()  [unwired: 1 in, 1 out]
        n94 = call "Console_Write.vi"("Code"="def testBLE():\n    try:\n        import ble_CBR\n        import ble_advertising\n        import ble_MIDI\n        print('BLE good')\n    except:\n        print('BLE bad')\n        \ntestBLE()\n", "Queue in"=w131) -> ()  [unwired: 10 in]
      }
      event "CtrlE": Value Change {
        # "Run code in CtrlE mode"
        n95 = event-data() -> ()  [unwired: 1 in, 1 out]
        n96 = call "Console_Run.vi"("Code"=w133, "Queue in"=w134) -> ()  [unwired: 10 in]
      }
      event "Spike": Value Change {
        # "Save file on SPIKE"
        n97 = event-data() -> ()  [unwired: 1 in, 1 out]
        n98 = call "Console_SaveFile.vi"("Path"=w135, "Code"=w136, "Queue in"=w137) -> ()  [unwired: 9 in]
      }
      event "reconnect": Value Change {
        # "Reconnect to SPIKE"
        n99 = event-data() -> ()  [unwired: 1 in, 1 out]
        n100 = call "Console_Reconnect.vi"("Queue in"=w138) -> ()  [unwired: 11 in]
      }
      event "Settings": Value Change {
        # "Edit settings"
        n101 = event-data() -> ()  [unwired: 1 in, 1 out]
        n102 = call "Preferences.vi"() -> ("Preferences out"=w139:T3)  [unwired: 10 in, 1 out]
        n103 = call "Settings.vi"("Prefs"=w139) -> ()  [unwired: 10 in, 1 out]
      }
      event "new lines": Value Change {
        # "update your plot"
        n104 = event-data() -> ()  [unwired: 1 in, 1 out]
        n105 = for {
          tunnel: "new lines" -> [w143] mode=indexing
          tunnel: w140 -> [w142]
          n106 = call "LsstLineDecode.vi"("new lines"=w143) -> ("Chart"=w146:dbl, "payload"=w144:string, "cmd"=w147:string, "Graph"=w145:dbl[])  [unwired: 6 in, 1 out]
          n107 = case shown="\"BLE\"" w147 {
            tunnel: w146 -> [w148 _ _ _ _]
            tunnel: w145 -> [_ w149 _ _ _]
            tunnel: w144 -> [_ _ w152 w159 _]
            tunnel: w142 -> [_ _ _ w156 _]
            frame "chart" {
              # "starts with a number"
              "Chart" <- w148
            }
            frame "graph" {
              # "starts with a bracket (array)"
              "Graph" <- w149
            }
            frame "version" {
              # "reply from version check"
              n108 = Equal?(x="good", y=w152) -> (x = y?=w150:bool)
              "good?" <- w150
              n109 = case shown="False" w150 {
                frame False {
                  n110 = One Button Dialog(message="SPIKE is not up to date! Please update SPIKE before continuing.", button name ("OK")="ok!") -> ()  [unwired: 1 out]
                }
                frame True {
                }
              }
            }
            frame "BLE" {
              n111 = Equal?(x="bad", y=w159) -> (x = y?=w157:bool)
              n112 = case shown="True" w157 {
                tunnel: w156 -> [_ w162]
                tunnel: [TRUE FALSE] -> w155
                frame False {
                }
                frame True {
                  n113 = call "uploadBLE.vi"("Queue in"=w162) -> ()  [unwired: 11 in]
                }
              }
              "BLE Good?" <- w155
            }
            frame Default {
              # "Some command"
            }
          }
        }
      }
    }
  }
  n114 = flat-sequence {
    tunnel: w2 -> [w166]
    tunnel: "Serial_Port" -> [w165]
    frame #0 {
      w164 = 1000  # Buffer Size
      # "Runs all things serial (the console).  Stops when you send stop on the queue"
      n115 = control-ref of="Console"() -> (w167:refnum<vi>)
      n116 = control-ref of="new lines"() -> (w163:refnum<vi>)
      n117 = call "Console.vi"("Buffer Size"=w164, "Last Lines"=w163, "Remote Console"=w167, "Queue in"=w166, "Python"=w165) -> ()  [unwired: 7 in]
    }
  }
